vi "Loop_SM.vi"() -> ()   [LabVIEW 2017, in "Gimbal.lvlib"]
uses:
  Gimbal.lvlib
  ENUM_SM_State.ctl
  ENUM_SM_Action.ctl
  Globals/Global_STOP.vi
  Global_CMD.vi
  Global_SM Write_Data Out.vi
panel:
  out "Input DBL Data":dbl
  out "Output Bool Data":bool
  out "Output DBL Data":dbl
  out "OutputI INT Data":i32
  out "Cycle Time (S)":dbl format="%.3g"
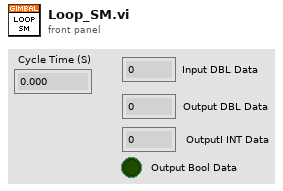
[diagram p1: front panel]
types:
  T1 = typedef "Gimbal.lvlib/ENUM_SM_State.ctl" = enum16{"Startup", "Idle", "Shutdown"}
  T2 = typedef "Gimbal.lvlib/ENUM_SM_Action.ctl" = enum16{"No Action", "Reset Time", "Reset All", "Action A", "Action B"}
  T3 = cluster{"State":T1, "Previous State":T1, "Current Time":timestamp, "Previous Time":timestamp, "Start Time":timestamp, "Target Time (ms)":u32, "Cycle Time(S)":dbl, "SM Input DBL":dbl, "SM Output DBL":dbl, "SM OutputI INT":i32, "SM Output Bool":bool}
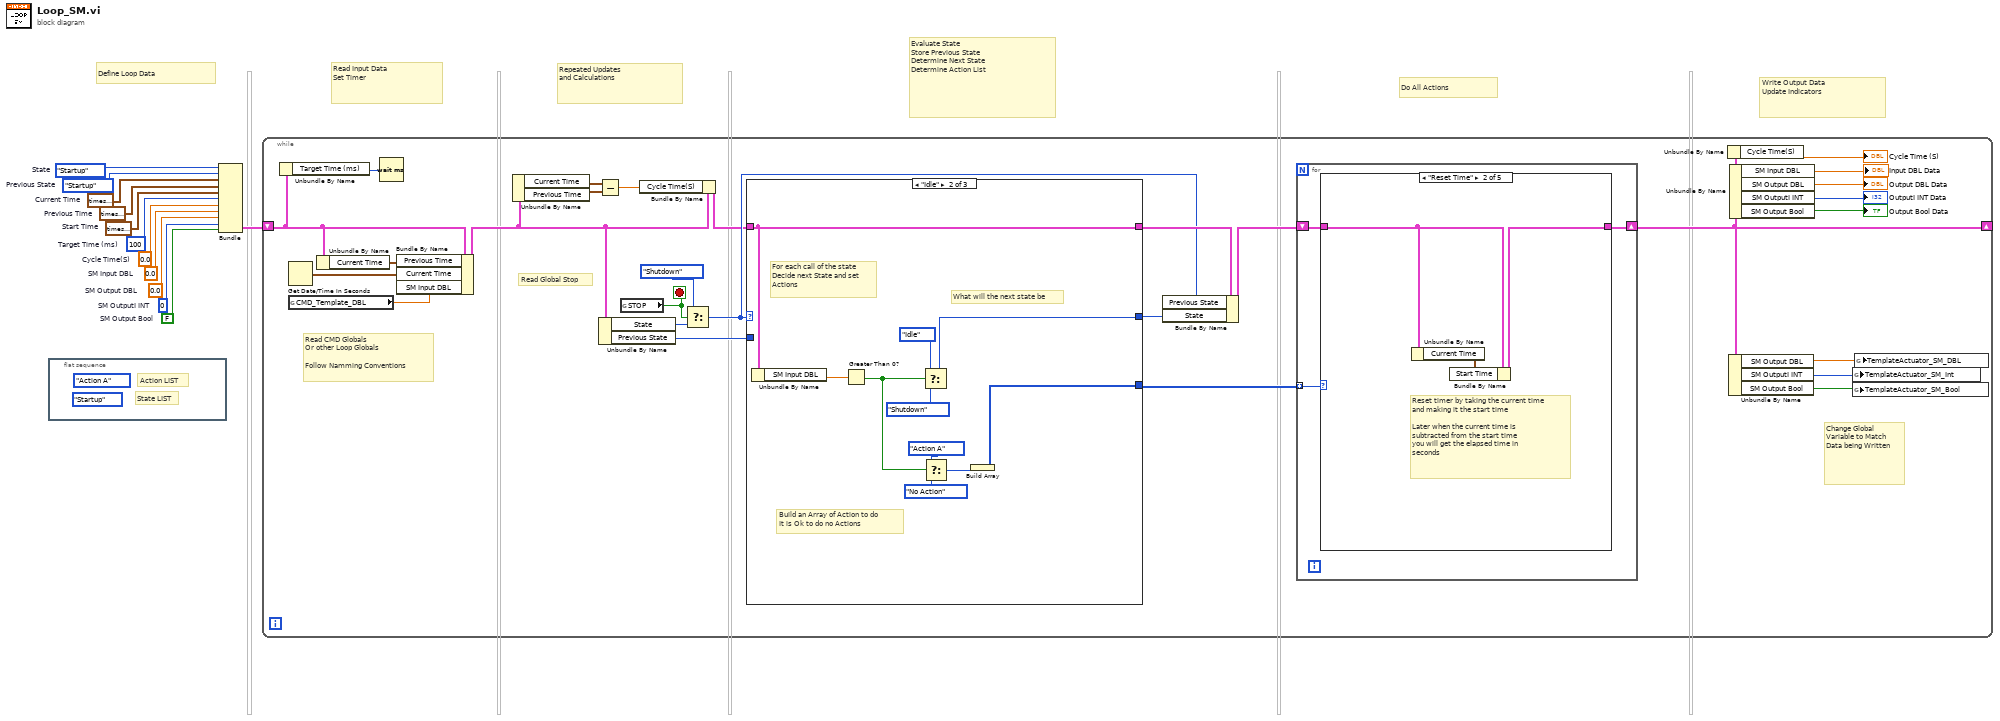
[diagram p0: block diagram]
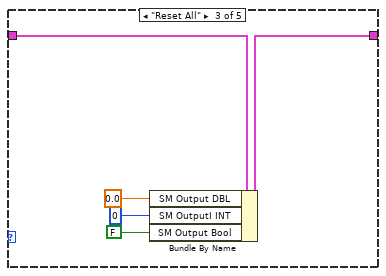
[diagram p3: hidden frame]
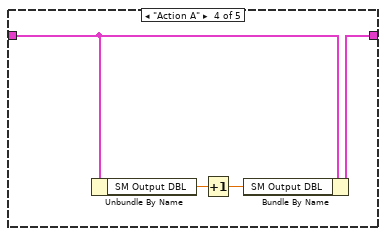
[diagram p4: hidden frame]
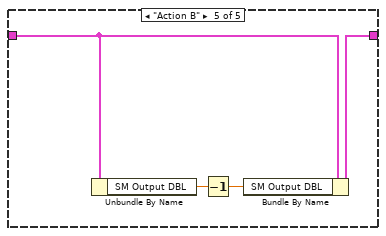
[diagram p5: hidden frame]
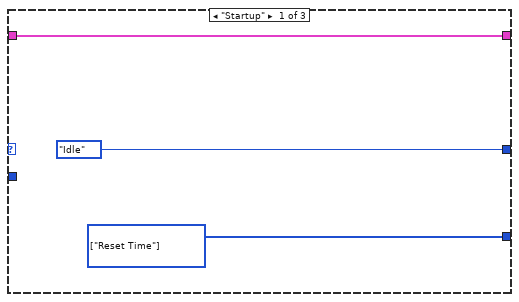
[diagram p6: hidden frame]
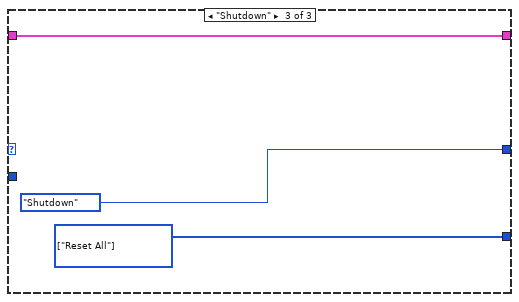
[diagram p7: hidden frame]
diagram:
  w1 = 0.0  # Cycle Time(S)
  w2 = ENUM_SM_State."Startup"  # Previous State
  w3 = timestamp(0 s since 1904-01-01)  # Previous Time
  w4 = FALSE  # SM Output Bool
  w5 = 0  # SM OutputI INT
  w6 = u32 100  # Target Time (ms)
  w7 = 0.0  # SM Output DBL
  w8 = 0.0  # SM Input DBL
  w9 = timestamp(0 s since 1904-01-01)  # Start Time
  w10 = timestamp(0 s since 1904-01-01)  # Current Time
  w11 = ENUM_SM_State."Startup"  # State
  # "Define Loop Data"
  # "Repeated Updates\nand Calculations"
  # "Read Input Data\nSet Timer"
  # "Evaluate State\nStore Previous State\nDetermine Next State\nDetermine Action List"
  # "Do All Actions"
  # "Write Output Data\nUpdate Indicators"
  n1 = flat-sequence {
    frame #0 {
      (unwired) ENUM_SM_State."Startup" ("State")
      (unwired) ENUM_SM_Action."Action A" ("Action")
      # "State LIST"
      # "Action LIST"
    }
  }
  n2 = Bundle("State"=w11, "Previous State"=w2, "Current Time"=w10, "Previous Time"=w3, "Start Time"=w9, "Target Time (ms)"=w6, "Cycle Time(S)"=w1, "SM Input DBL"=w8, "SM Output DBL"=w7, "SM OutputI INT"=w5, "SM Output Bool"=w4) -> (w12:T3)  [unwired: 1 in]
  n3 = while {
    shift-right: [w22] -> _
    shift-left: w12 -> [w28]
    stop <- w36 stop-if-true
    # "Change Global\nVariable to Match\nData being Written"
    # "Read CMD Globals\nOr other Loop Globals\n\nFollow Namming Conventions"
    # "Read Global Stop"
    n4 = Unbundle By Name(w28) -> ("Target Time (ms)"=w33:u32)
    n5 = Get Date/Time In Seconds() -> (seconds since 1Jan1904=w40:timestamp)
    n6 = global read "Global_CMD.vi" "CMD_Template_DBL"() -> (w13:dbl)
    n7 = Unbundle By Name(w28) -> ("Current Time"=w29:timestamp)
    n8 = Wait (ms)(milliseconds to wait=w33) -> ()  [unwired: 1 out]
    n9 = Bundle By Name(cluster=w28, "Previous Time"=w29, "Current Time"=w40, "SM Input DBL"=w13) -> (w18:T3)
    n10 = Unbundle By Name(w18) -> ("Current Time"=w19:timestamp, "Previous Time"=w20:timestamp)
    n11 = Subtract(x=w19, y=w20) -> (x-y=w16:dbl)
    n12 = Unbundle By Name(w18) -> ("State"=w34:T1, "Previous State"=w27:T1)
    n13 = global read "Global_STOP.vi" "STOP"() -> (w36:bool)
    n14 = Bundle By Name(cluster=w18, "Cycle Time(S)"=w16) -> (w17:T3)
    n15 = Select(t=ENUM_SM_State."Shutdown" ("State"), s=w36, f=w34) -> (s? t:f=w23:T1)
    n16 = case shown="\"Idle\"" w23 {
      tunnel: w17 -> [w63 w73 w76]
      tunnel: [w63 w73 w76] -> w38
      tunnel: [ENUM_SM_State."Idle" ("State") w71 ENUM_SM_State."Shutdown" ("State")] -> w37
      tunnel: [w62 w64 w74] -> w15
      tunnel: w27 -> [_ _ _]
      frame "Startup" {
        w62 = T2[] [enum."Reset Time"] items=["No Action", "Reset Time", "Reset All", "Action A", "Action B"] ("Actions")
      }
      frame "Idle" {
        # "For each call of the state\nDecide next State and set\nActions"
        # "What will the next state be"
        # "Build an Array of Action to do\nIt is Ok to do no Actions"
        n17 = Unbundle By Name(w73) -> ("SM Input DBL"=w72:dbl)
        n18 = Greater Than 0?(x=w72) -> (x > 0?=w66:bool)
        n19 = Select(t=ENUM_SM_State."Idle" ("State"), s=w66, f=ENUM_SM_State."Shutdown" ("State")) -> (s? t:f=w71:T1)
        n20 = Select(t=ENUM_SM_Action."Action A" ("Action"), s=w66, f=ENUM_SM_Action."No Action" ("Action")) -> (s? t:f=w65:T2)
        n21 = Build Array(w65) -> (w64:T2[])
      }
      frame "Shutdown" {
        w74 = T2[] [enum."Reset All"] items=["No Action", "Reset Time", "Reset All", "Action A", "Action B"] ("Actions")
      }
    }
    n22 = Bundle By Name(cluster=w38, "Previous State"=w23, "State"=w37) -> (w39:T3)
    n23 = for {
      tunnel: w15 -> [w43] mode=indexing
      shift-right: [w42] -> w22
      shift-left: w39 -> [w41]
      n24 = case shown="\"Reset Time\"" w43 {
        tunnel: w41 -> [w44 w47 w52 w55 w59]
        tunnel: [w44 w46 w51 w54 w58] -> w42
        frame "No Action" {
        }
        frame "Reset Time" {
          # "Reset timer by taking the current time\nand making it the start time\n\nLater when the current time is \nsubtracted from the start time\nyou will get the elapsed time in \nseconds"
          n25 = Unbundle By Name(w47) -> ("Current Time"=w45:timestamp)
          n26 = Bundle By Name(cluster=w47, "Start Time"=w45) -> (w46:T3)
        }
        frame "Reset All" {
          n27 = Bundle By Name(cluster=w52, "SM Output DBL"=0.0 ("FG Write Value"), "SM OutputI INT"=0 ("OutputI INT"), "SM Output Bool"=FALSE ("Output Bool")) -> (w51:T3)
        }
        frame "Action A" {
          n28 = Unbundle By Name(w55) -> ("SM Output DBL"=w56:dbl)
          n29 = Increment(x=w56) -> (x+1=w53:dbl)
          n30 = Bundle By Name(cluster=w55, "SM Output DBL"=w53) -> (w54:T3)
        }
        frame "Action B" {
          n31 = Unbundle By Name(w59) -> ("SM Output DBL"=w60:dbl)
          n32 = Decrement(x=w60) -> (x-1=w57:dbl)
          n33 = Bundle By Name(cluster=w59, "SM Output DBL"=w57) -> (w58:T3)
        }
      }
    }
    n34 = Unbundle By Name(w22) -> ("Cycle Time(S)"=→"Cycle Time (S)":dbl)
    n35 = Unbundle By Name(w22) -> ("SM Output DBL"=w30:dbl, "SM OutputI INT"=w31:i32, "SM Output Bool"=w32:bool)
    n36 = Unbundle By Name(w22) -> ("SM Input DBL"=→"Input DBL Data":dbl, "SM Output DBL"=→"Output DBL Data":dbl, "SM OutputI INT"=→"OutputI INT Data":i32, "SM Output Bool"=→"Output Bool Data":bool)
    n37 = global write "Global_SM Write_Data Out.vi" "TemplateActuator_SM_Int"(w31) -> ()
    n38 = global write "Global_SM Write_Data Out.vi" "TemplateActuator_SM_Bool"(w32) -> ()
    n39 = global write "Global_SM Write_Data Out.vi" "TemplateActuator_SM_DBL"(w30) -> ()
  }
